vi "Close.vi"(8 "error in (no error)":errorcluster, 11 "TcpSocket in":refnum<class "TcpSocket.lvclass">) -> (0 "error out":errorcluster)   [LabVIEW 2022 SP3, in "TcpSocket.lvlib" / "TcpSocket.lvclass"]
uses:
  TcpSocket.lvclass
  TcpSocket.lvclass/TcpSocket.ctl
  Read Connection.vi
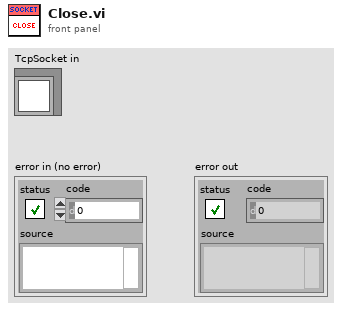
[diagram p1: front panel]
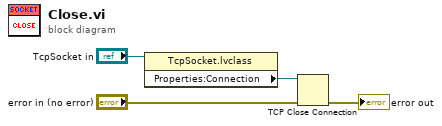
[diagram p0: block diagram]
diagram:
  n1 = property class="TcpSocket.lvclass"(reference="TcpSocket in") -> ("Properties:Connection"=w4:refnum<k5>)  [unwired: 1 in, 2 out]
  n2 = TCP Close Connection(connection ID=w4, error in (no error)="error in (no error)") -> (error out=→"error out":errorcluster)  [unwired: 1 in, 1 out]
